vi "Update JSON Config Req.vi"(8 "error in (no error)":errorcluster, 10 "ConfigRequest":T1={"SMUResourceName"="SMU1", "SMUChannels"="0:1", "SMUSourceMode"=1022, "SMUOutputFunction"=1008, "SMUSourceTransientResponse"=1040, "SMUCurrent"=2.0, "SMUCurrentLevelRange"=2.0, "SMUMeasurementSense"=1009, "SMUMeasurementApertureTime"=0.011, "SMUSourceAdvancedSourceDelay"=0.000101, "SMUVoltage"=7.0, "SMUSourceAdvancedSequenceLoopCount"=701, "SMUMeasurementAdvancedDCNoiseRejection"=1045, "SMUSequenceName"="YourSequence", "ScanList"="", "DMMResourceName"="DMM1", "DMMFunction"=1, "DMMResolution"=0.2, "DMMRange"=0.2, "DMMSampleCount"=1, "DMMApertureTimeUnit"=1, "DMMApertureTime"=0.011, "DMMNumberOfAverages"=2, "DMMAutoZero"=1, "DMMADCCalibration"=1, "DMMSettleTime"=0.0002, "DMMControlAction"=1, "DMMVoltageFaultUpperLimit"=5.1e-05, "ApplicationNumberOfWeldChannels"=8}, 11 "JSON Configuration File (.json)":path=path "C:/Users/chericks/Desktop/JSONfun/jsonbefore.json") -> (0 "error out":errorcluster)   [LabVIEW 2019]
uses:
  JSONCluster.ctl
  labview-grpc-query-server/VIs/MeasurementServer_ConfigRequest.ctl
  labview-grpc-query-server/VIs/labview-grpc-measurement-server.lvlib
panel:
  out "File Contents":string="{\n    \"SMUResourceName\": \"SMU\",\n    \"SMUChannels\": \"0\",\n\t\"SMUSourceMode\": 1021,\n\t\"SMUOutputFunction\": 1007,\n    \"SMUSourceTransientResponse\": 1039,\n    \"SMUCurrent\": 1.0,\n    \"SMUCurrentLevelRange\": 1.0,\n    \"SMUMeasurementSense\": 1008,\n    \"SMUMeasurementApertureTime\": 0.010,\n    \"SMUSourceAdvancedSourceDelay\": 0.000100,\n    \"SMUVoltage\": 6,\n    \"SMUSourceAdvancedSequenceLoopCount\": 700,\n    \"SMUMeasurementAdvancedDCNoiseRejection\": 1044,\n\t\"SMUSequenceName\": \"MySequence\",\n\t\"SMUStep1_Source_DCCurrent_CurrentLevel\": 1150009,\n\t\"SMUStep2_Measurement_ApertureTime\": 1150058,\n\t\"SMUStep3_Source_Advanced_SourceDelay\": 1150051,\n\t\"SMUSequenceNumberOfSteps\": 3,\n\t\t\n\t\"Switch1ResourceName\": \"2526_1\",\n\t\"Switch1Topology\": \"2526/2-Wire 79x1 Mux\",\n\t\"Switch1ScanList\": \"ch70:76->com\",\n\t\n\t\"Switch2ResourceName\": \"SwitchBlock1Dev1\",\n\t\"Switch2Topology\": \"Configured Topology\",\n\t\"Switch2ScanList\": \"[c2->card1r2->c26], [c3->card1r3->c27]; [c6->card1r2->c26], [c7->card1r3->c27]; [c10->card1r2->c26], [c11->card1r3->c27]; [c14->card1r2->c26], [c15->card1r3->c27]; [c18->card1r2->c26], [c19->card1r3->c27]; [c22->card1r2->c26], [c23->card1r3->c27]; [c30->card1r2->c26], [c31->card1r3->c27];\",\n\t\n\t\"DMMResourceName\": \"DMM\",\n\t\"DMMFunction\": 0,\n\t\"DMMResolution\": 0.1,\n\t\"DMMRange\": 0.1,\n\t\"DMMSampleCount\": 0,\n\t\"DMMApertureTimeUnit\": 0,\n\t\"DMMApertureTime\": 0.010,\n\t\"DMMNumberOfAverages\": 1,\n\t\"DMMAutoZero\": 0,\n\t\"DMMADCCalibration\": 0,\n\t\"DMMSettleTime\": 0.0001,\n\t\"DMMControlAction\": 0,\n\t\"DMMVoltageFaultUpperLimit\": 0.000050,\n\t\n\t\"ApplicationNumberOfWeldChannels\": 7\n}"
  out "JSONCluster":T2={"SMUResourceName"="SMU", "SMUChannels"="0", "SMUSourceMode"=1021, "SMUOutputFunction"=1007, "SMUSourceTransientResponse"=1039, "SMUCurrent"=1.0, "SMUCurrentLevelRange"=1.0, "SMUMeasurementSense"=1008, "SMUMeasurementApertureTime"=0.01, "SMUSourceAdvancedSourceDelay"=0.0001, "SMUVoltage"=6.0, "SMUSourceAdvancedSequenceLoopCount"=700, "SMUMeasurementAdvancedDCNoiseRejection"=1044, "SMUSequenceName"="MySequence", "SMUStep1_Source_DCCurrent_CurrentLevel"=1150009, "SMUStep2_Measurement_ApertureTime"=1150058, "SMUStep3_Source_Advanced_SourceDelay"=1150051, "SMUSequenceNumberOfSteps"=3, "ScanList"="", "Switch1ResourceName"="2526_1", "Switch1Topology"="2526/2-Wire 79x1 Mux", "Switch1ScanList"="ch70:76->com", "Switch2ResourceName"="SwitchBlock1Dev1", "Switch2Topology"="Configured Topology", "Switch2ScanList"="[c2->card1r2->c26], [c3->card1r3->c27]; [c6->card1r2->c26], [c7->card1r3->c27]; [c10->card1r2->c26], [c11->card1r3->c27]; [c14->card1r2->c26], [c15->card1r3->c27]; [c18->card1r2->c26], [c19->card1r3->c27]; [c22->card1r2->c26], [c23->card1r3->c27]; [c30->card1r2->c26], [c31->card1r3->c27];", "DMMResourceName"="DMM", "DMMFunction"=0, "DMMResolution"=0.1, "DMMRange"=0.1, "DMMSampleCount"=0, "DMMApertureTimeUnit"=0, "DMMApertureTime"=0.01, "DMMNumberOfAverages"=1, "DMMAutoZero"=0, "DMMADCCalibration"=0, "DMMSettleTime"=0.0001, "DMMControlAction"=0, "DMMVoltageFaultUpperLimit"=5e-05, "ApplicationNumberOfWeldChannels"=7}
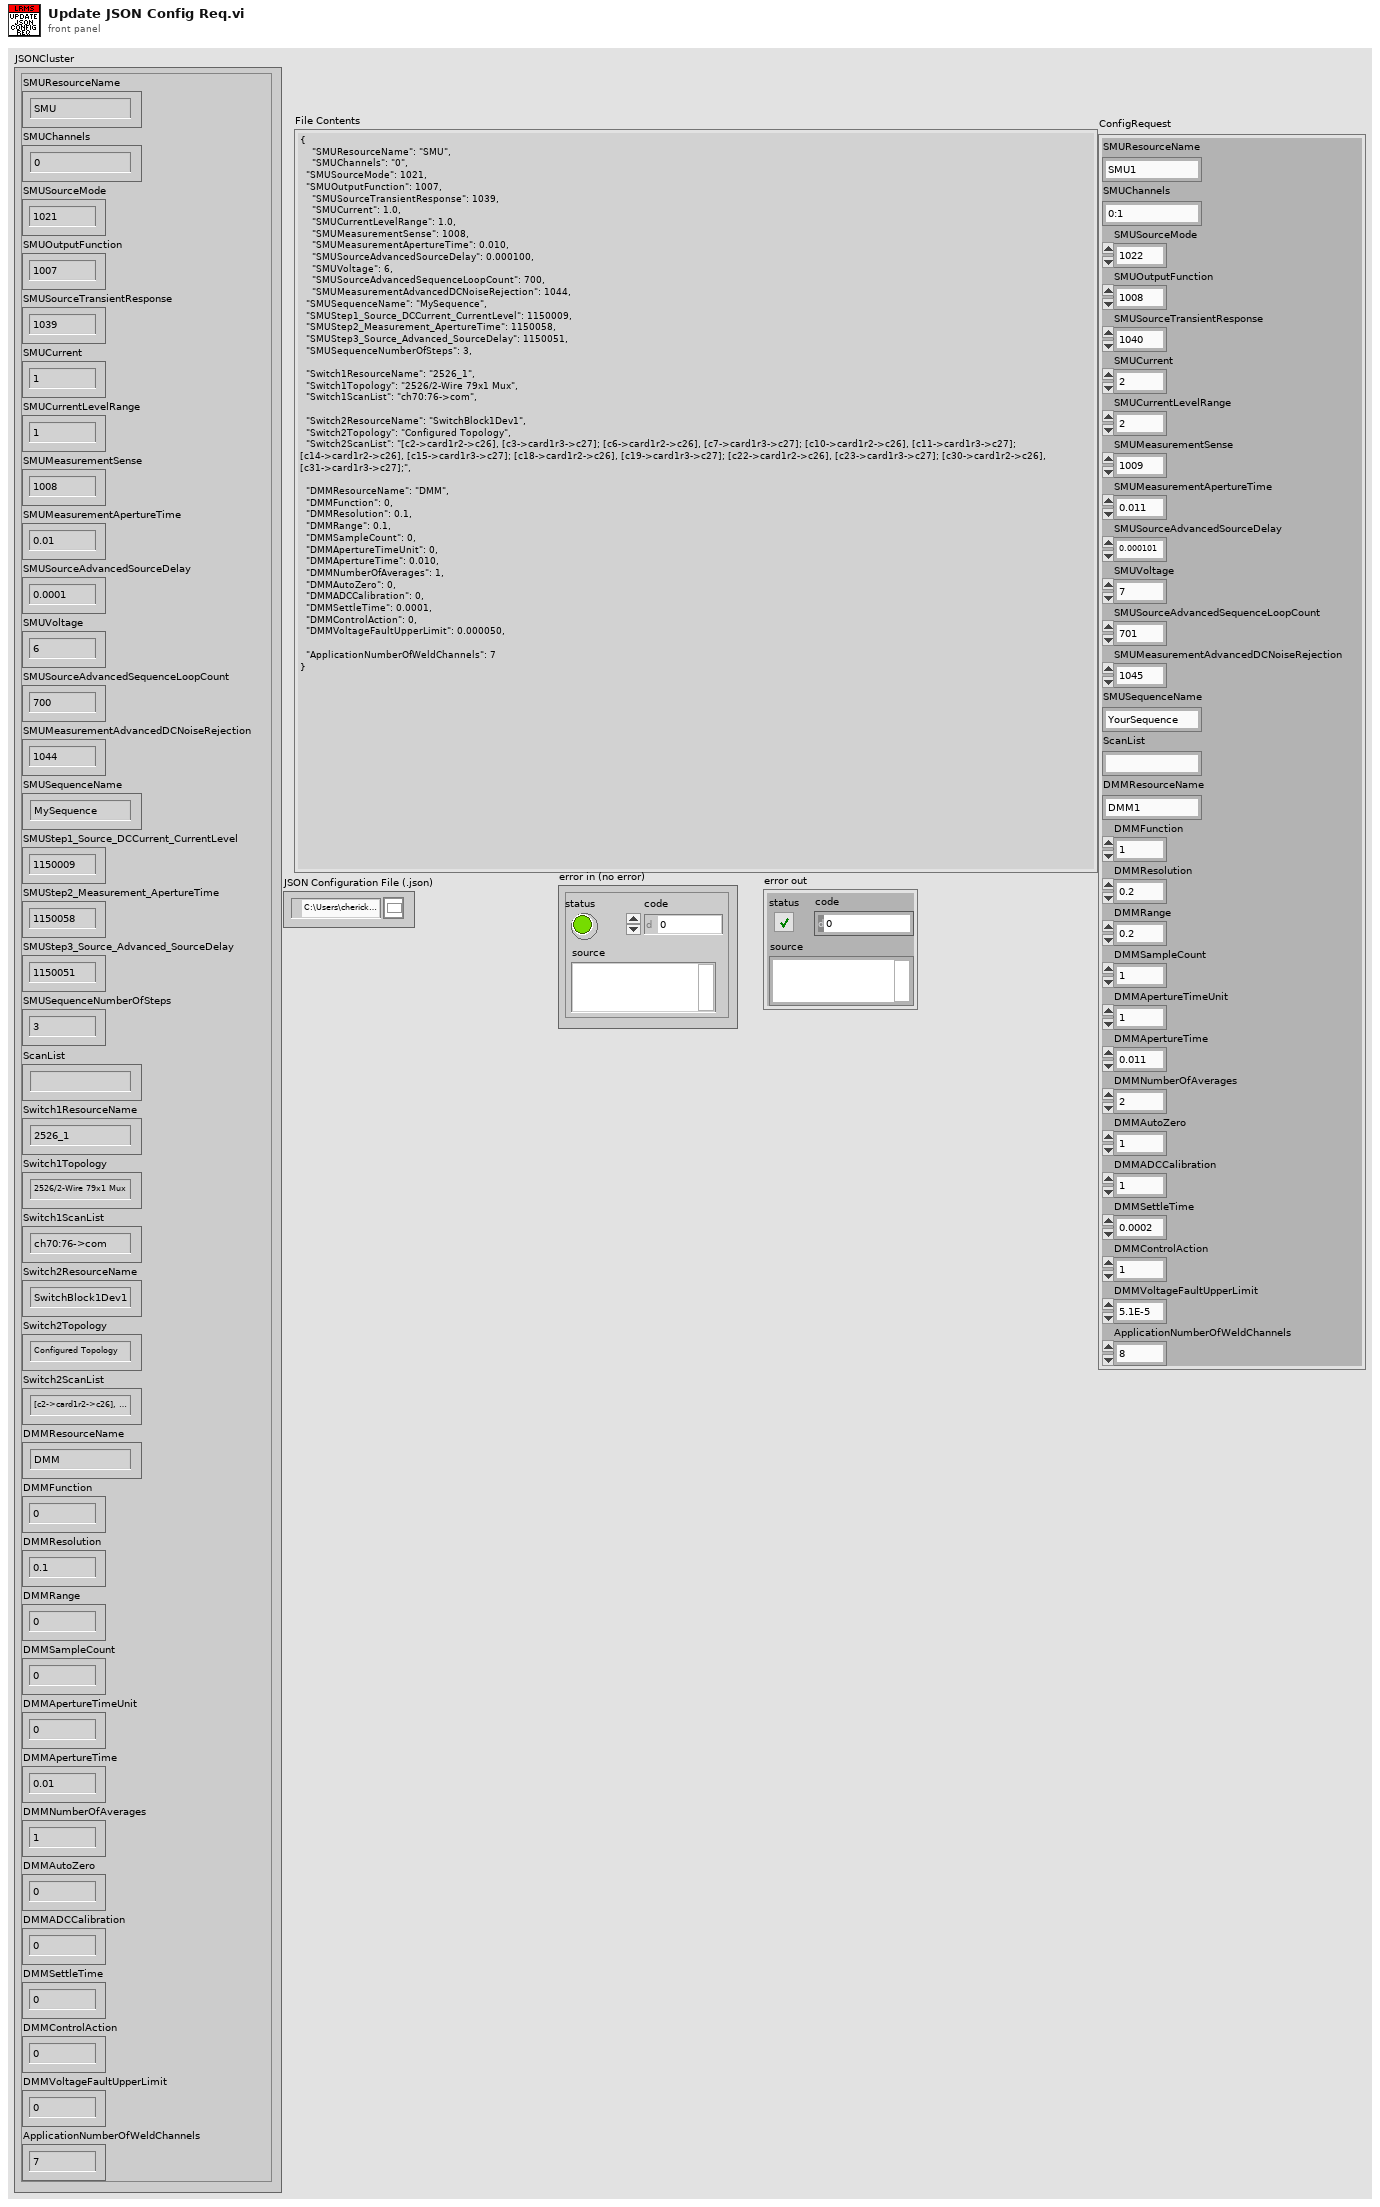
[diagram p1: front panel]
types:
  T1 = typedef "labview-grpc-measurement-server.lvlib/MeasurementServer_ConfigRequest.ctl" = cluster{"SMUResourceName":string, "SMUChannels":string, "SMUSourceMode":i32, "SMUOutputFunction":i32, "SMUSourceTransientResponse":i32, "SMUCurrent":sgl, "SMUCurrentLevelRange":sgl, "SMUMeasurementSense":i32, "SMUMeasurementApertureTime":sgl, "SMUSourceAdvancedSourceDelay":sgl, "SMUVoltage":sgl, "SMUSourceAdvancedSequenceLoopCount":i32, "SMUMeasurementAdvancedDCNoiseRejection":i32, "SMUSequenceName":string, "ScanList":string, "DMMResourceName":string, "DMMFunction":i32, "DMMResolution":sgl, "DMMRange":sgl, "DMMSampleCount":i32, "DMMApertureTimeUnit":i32, "DMMApertureTime":sgl, "DMMNumberOfAverages":i32, "DMMAutoZero":i32, "DMMADCCalibration":i32, "DMMSettleTime":sgl, "DMMControlAction":i32, "DMMVoltageFaultUpperLimit":sgl, "ApplicationNumberOfWeldChannels":i32}
  T2 = typedef "JSONCluster.ctl" = cluster{"SMUResourceName":string, "SMUChannels":string, "SMUSourceMode":i32, "SMUOutputFunction":i32, "SMUSourceTransientResponse":i32, "SMUCurrent":dbl, "SMUCurrentLevelRange":dbl, "SMUMeasurementSense":i32, "SMUMeasurementApertureTime":dbl, "SMUSourceAdvancedSourceDelay":dbl, "SMUVoltage":dbl, "SMUSourceAdvancedSequenceLoopCount":i32, "SMUMeasurementAdvancedDCNoiseRejection":i32, "SMUSequenceName":string, "SMUStep1_Source_DCCurrent_CurrentLevel":i32, "SMUStep2_Measurement_ApertureTime":i32, "SMUStep3_Source_Advanced_SourceDelay":i32, "SMUSequenceNumberOfSteps":i32, "ScanList":string, "Switch1ResourceName":string, "Switch1Topology":string, "Switch1ScanList":string, "Switch2ResourceName":string, "Switch2Topology":string, "Switch2ScanList":string, "DMMResourceName":string, "DMMFunction":i32, "DMMResolution":dbl, "DMMRange":dbl, "DMMSampleCount":i32, "DMMApertureTimeUnit":i32, "DMMApertureTime":dbl, "DMMNumberOfAverages":i32, "DMMAutoZero":i32, "DMMADCCalibration":i32, "DMMSettleTime":dbl, "DMMControlAction":i32, "DMMVoltageFaultUpperLimit":dbl, "ApplicationNumberOfWeldChannels":i32}
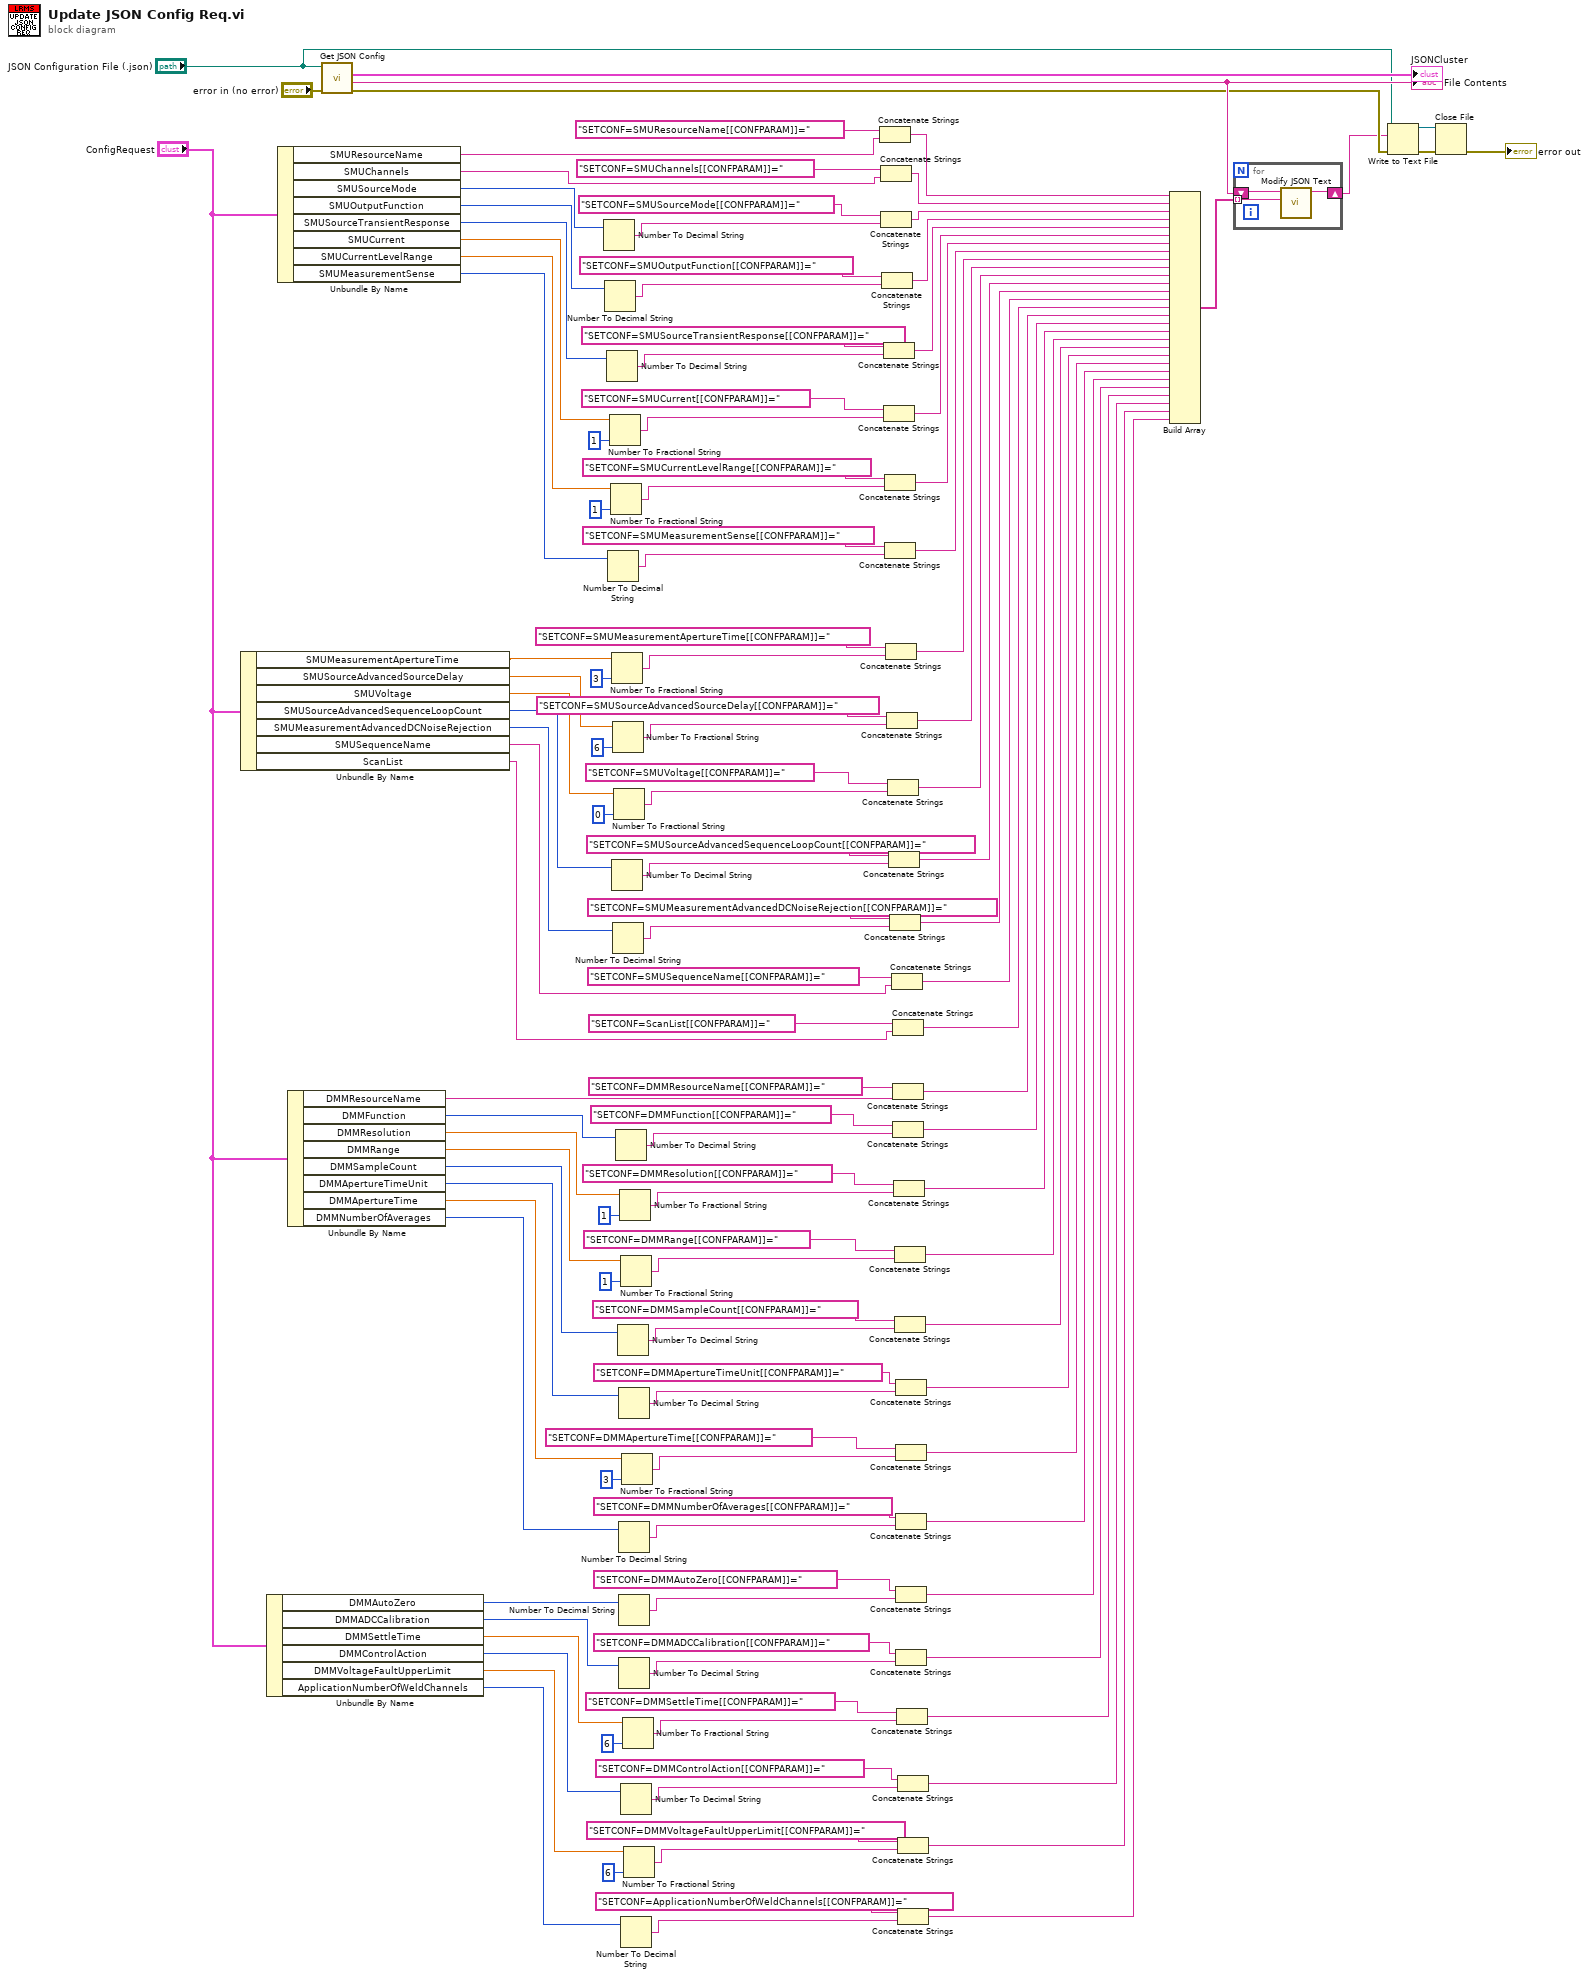
[diagram p0: block diagram]
diagram:
  n1 = Unbundle By Name("ConfigRequest") -> ("SMUMeasurementApertureTime"=w86:sgl, "SMUSourceAdvancedSourceDelay"=w85:sgl, "SMUVoltage"=w79:sgl, "SMUSourceAdvancedSequenceLoopCount"=w75:i32, "SMUMeasurementAdvancedDCNoiseRejection"=w71:i32, "SMUSequenceName"=w68:string, "ScanList"=w65:string)
  n2 = Unbundle By Name("ConfigRequest") -> ("DMMAutoZero"=w27:i32, "DMMADCCalibration"=w23:i32, "DMMSettleTime"=w19:sgl, "DMMControlAction"=w14:i32, "DMMVoltageFaultUpperLimit"=w9:sgl, "ApplicationNumberOfWeldChannels"=w5:i32)
  n3 = Unbundle By Name("ConfigRequest") -> ("SMUResourceName"=w130:string, "SMUChannels"=w127:string, "SMUSourceMode"=w118:i32, "SMUOutputFunction"=w112:i32, "SMUSourceTransientResponse"=w108:i32, "SMUCurrent"=w105:sgl, "SMUCurrentLevelRange"=w98:sgl, "SMUMeasurementSense"=w94:i32)
  n4 = Unbundle By Name("ConfigRequest") -> ("DMMResourceName"=w63:string, "DMMFunction"=w59:i32, "DMMResolution"=w54:sgl, "DMMRange"=w50:sgl, "DMMSampleCount"=w45:i32, "DMMApertureTimeUnit"=w42:i32, "DMMApertureTime"=w36:sgl, "DMMNumberOfAverages"=w32:i32)
  n5 = call "Get JSON Config.vi"("error in (no error)"="error in (no error)", "JSON Configuration File (.json)"="JSON Configuration File (.json)") -> ("error out"=w120:errorcluster, "File Contents"=w129:string, "JSONCluster"=→"JSONCluster":T2)  [unwired: 6 in, 1 out]
  "File Contents" <- w129
  n6 = Number To Decimal String(number=w118) -> (decimal integer string=w116:string)  [unwired: 1 in]
  n7 = Number To Decimal String(number=w112) -> (decimal integer string=w113:string)  [unwired: 1 in]
  n8 = Number To Decimal String(number=w108) -> (decimal integer string=w109:string)  [unwired: 1 in]
  n9 = Number To Decimal String(number=w94) -> (decimal integer string=w95:string)  [unwired: 1 in]
  n10 = Number To Fractional String(number=w105, precision (6)=i16 1) -> (F-format string=w104:string)  [unwired: 2 in]
  n11 = Number To Fractional String(number=w98, precision (6)=i16 1) -> (F-format string=w100:string)  [unwired: 2 in]
  n12 = Number To Fractional String(number=w86, precision (6)=i16 3) -> (F-format string=w91:string)  [unwired: 2 in]
  n13 = Number To Decimal String(number=w75) -> (decimal integer string=w76:string)  [unwired: 1 in]
  n14 = Number To Fractional String(number=w85, precision (6)=i16 6) -> (F-format string=w88:string)  [unwired: 2 in]
  n15 = Number To Decimal String(number=w71) -> (decimal integer string=w72:string)  [unwired: 1 in]
  n16 = Number To Fractional String(number=w79, precision (6)=i16 0) -> (F-format string=w81:string)  [unwired: 2 in]
  n17 = Number To Decimal String(number=w59) -> (decimal integer string=w60:string)  [unwired: 1 in]
  n18 = Number To Decimal String(number=w45) -> (decimal integer string=w46:string)  [unwired: 1 in]
  n19 = Number To Decimal String(number=w42) -> (decimal integer string=w43:string)  [unwired: 1 in]
  n20 = Number To Decimal String(number=w32) -> (decimal integer string=w34:string)  [unwired: 1 in]
  n21 = Number To Decimal String(number=w27) -> (decimal integer string=w29:string)  [unwired: 1 in]
  n22 = Number To Decimal String(number=w23) -> (decimal integer string=w25:string)  [unwired: 1 in]
  n23 = Number To Fractional String(number=w54, precision (6)=i16 1) -> (F-format string=w56:string)  [unwired: 2 in]
  n24 = Number To Fractional String(number=w50, precision (6)=i16 1) -> (F-format string=w52:string)  [unwired: 2 in]
  n25 = Number To Decimal String(number=w14) -> (decimal integer string=w16:string)  [unwired: 1 in]
  n26 = Number To Decimal String(number=w5) -> (decimal integer string=w7:string)  [unwired: 1 in]
  n27 = Number To Fractional String(number=w36, precision (6)=i16 3) -> (F-format string=w38:string)  [unwired: 2 in]
  n28 = Number To Fractional String(number=w19, precision (6)=i16 6) -> (F-format string=w21:string)  [unwired: 2 in]
  n29 = Number To Fractional String(number=w9, precision (6)=i16 6) -> (F-format string=w12:string)  [unwired: 2 in]
  n30 = Concatenate Strings("SETCONF=SMUResourceName[[CONFPARAM]]=", w130) -> (w128:string)
  n31 = Concatenate Strings("SETCONF=SMUChannels[[CONFPARAM]]=", w127) -> (w125:string)
  n32 = Concatenate Strings("SETCONF=SMUSourceMode[[CONFPARAM]]=", w116) -> (w115:string)
  n33 = Concatenate Strings("SETCONF=SMUOutputFunction[[CONFPARAM]]=", w113) -> (w111:string)
  n34 = Concatenate Strings("SETCONF=SMUSourceTransientResponse[[CONFPARAM]]=", w109) -> (w107:string)
  n35 = Concatenate Strings("SETCONF=SMUCurrent[[CONFPARAM]]=", w104) -> (w103:string)
  n36 = Concatenate Strings("SETCONF=SMUCurrentLevelRange[[CONFPARAM]]=", w100) -> (w97:string)
  n37 = Concatenate Strings("SETCONF=SMUMeasurementSense[[CONFPARAM]]=", w95) -> (w93:string)
  n38 = Concatenate Strings("SETCONF=SMUMeasurementApertureTime[[CONFPARAM]]=", w91) -> (w84:string)
  n39 = Concatenate Strings("SETCONF=SMUSourceAdvancedSourceDelay[[CONFPARAM]]=", w88) -> (w83:string)
  n40 = Concatenate Strings("SETCONF=SMUVoltage[[CONFPARAM]]=", w81) -> (w78:string)
  n41 = Concatenate Strings("SETCONF=SMUSourceAdvancedSequenceLoopCount[[CONFPARAM]]=", w76) -> (w74:string)
  n42 = Concatenate Strings("SETCONF=SMUMeasurementAdvancedDCNoiseRejection[[CONFPARAM]]=", w72) -> (w70:string)
  n43 = Concatenate Strings("SETCONF=SMUSequenceName[[CONFPARAM]]=", w68) -> (w67:string)
  n44 = Concatenate Strings("SETCONF=ScanList[[CONFPARAM]]=", w65) -> (w1:string)
  n45 = Concatenate Strings("SETCONF=DMMResourceName[[CONFPARAM]]=", w63) -> (w62:string)
  n46 = Concatenate Strings("SETCONF=DMMFunction[[CONFPARAM]]=", w60) -> (w58:string)
  n47 = Concatenate Strings("SETCONF=DMMResolution[[CONFPARAM]]=", w56) -> (w53:string)
  n48 = Concatenate Strings("SETCONF=DMMRange[[CONFPARAM]]=", w52) -> (w48:string)
  n49 = Concatenate Strings("SETCONF=DMMSampleCount[[CONFPARAM]]=", w46) -> (w44:string)
  n50 = Concatenate Strings("SETCONF=DMMApertureTimeUnit[[CONFPARAM]]=", w43) -> (w40:string)
  n51 = Concatenate Strings("SETCONF=DMMApertureTime[[CONFPARAM]]=", w38) -> (w35:string)
  n52 = Concatenate Strings("SETCONF=DMMNumberOfAverages[[CONFPARAM]]=", w34) -> (w31:string)
  n53 = Concatenate Strings("SETCONF=DMMAutoZero[[CONFPARAM]]=", w29) -> (w26:string)
  n54 = Concatenate Strings("SETCONF=DMMADCCalibration[[CONFPARAM]]=", w25) -> (w22:string)
  n55 = Concatenate Strings("SETCONF=DMMSettleTime[[CONFPARAM]]=", w21) -> (w17:string)
  n56 = Concatenate Strings("SETCONF=DMMControlAction[[CONFPARAM]]=", w16) -> (w13:string)
  n57 = Concatenate Strings("SETCONF=DMMVoltageFaultUpperLimit[[CONFPARAM]]=", w12) -> (w8:string)
  n58 = Concatenate Strings("SETCONF=ApplicationNumberOfWeldChannels[[CONFPARAM]]=", w7) -> (w4:string)
  n59 = Build Array(w128, w125, w115, w111, w107, w103, w97, w93, w84, w83, w78, w74, w70, w67, w1, w62, w58, w53, w48, w44, w40, w35, w31, w26, w22, w17, w13, w8, w4) -> (w124:string[])
  n60 = for {
    tunnel: w124 -> [w135] mode=indexing
    shift-right: [w134] -> w119
    shift-left: w129 -> [w133]
    n61 = call "Modify JSON Text.vi"("Parameter and Value"=w135, "JSONtextin"=w133) -> ("JSONtextout"=w134:string)  [unwired: 9 in]
  }
  n62 = Write to Text File(file (use dialog)="JSON Configuration File (.json)", text=w119, error in=w120) -> (refnum out=w123:refnum<file>, error out=w122:errorcluster)  [unwired: 1 in, 1 out]
  n63 = Close File(refnum=w123, error in=w122) -> (error out=→"error out":errorcluster)  [unwired: 1 out]
